vi "Atoi, four scalars.vi"(4 "string 4":string, 5 "string 3":string, 6 "string 2":string, 7 "string 1":string) -> (0 "number 4":i32, 1 "number 3":i32, 2 "number 2":i32, 3 "number 1":i32)   [LabVIEW 2010]
doc: "Converts four strings to four signed integers (with rounding)."
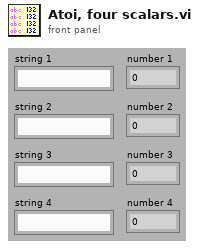
[diagram p1: front panel]
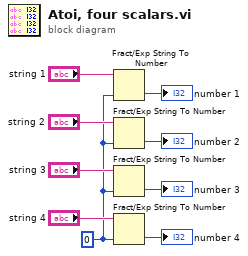
[diagram p0: block diagram]
diagram:
  w1 = 0 ("Result")
  n1 = Fract/Exp String To Number(string="string 1", default (0 dbl)=w1) -> (number=→"number 1":i32)  [unwired: 2 in, 1 out]
  n2 = Fract/Exp String To Number(string="string 2", default (0 dbl)=w1) -> (number=→"number 2":i32)  [unwired: 2 in, 1 out]
  n3 = Fract/Exp String To Number(string="string 3", default (0 dbl)=w1) -> (number=→"number 3":i32)  [unwired: 2 in, 1 out]
  n4 = Fract/Exp String To Number(string="string 4", default (0 dbl)=w1) -> (number=→"number 4":i32)  [unwired: 2 in, 1 out]
